vi "Read Parameter Spreadsheet.vi"(8 "error in (no error)":errorcluster) -> (0 "error out":errorcluster, 1 "Constraints":string[](array[string]), 2 "Types":string[](array[string]), 3 "Names":string[](array[string]), 5 "EnumVals":i32[](array[numeric]))   [LabVIEW 2020, in "Camera.lvlib"]
uses:
  Camera.lvlib
  <vilib>/Utility/file.llb/Read Delimited Spreadsheet (string).vi
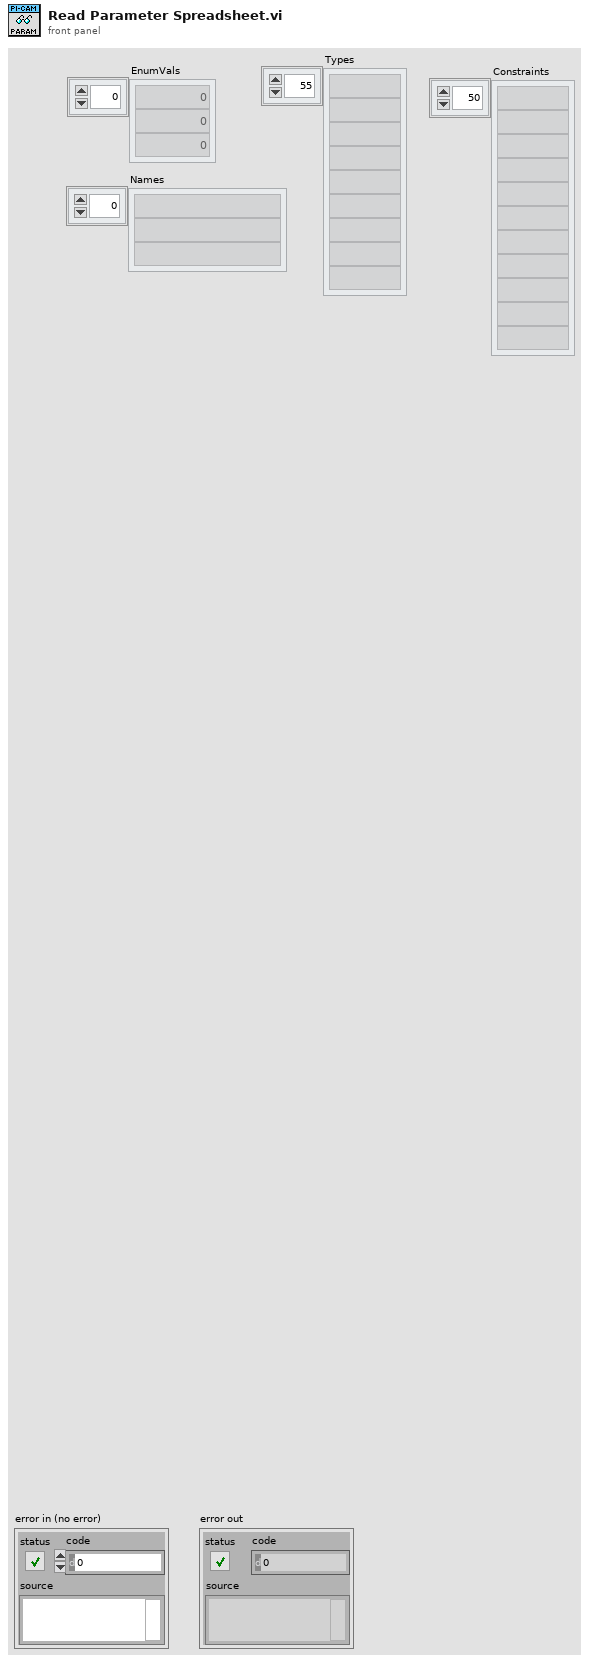
[diagram p1: front panel]
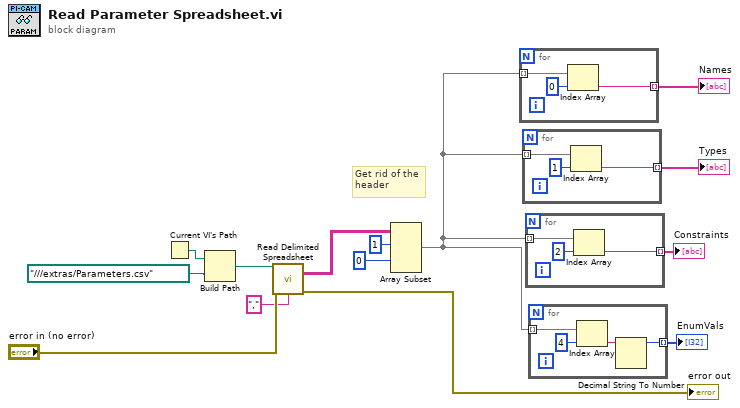
[diagram p0: block diagram]
diagram:
  # "Get rid of the\nheader"
  n1 = Current VI's Path() -> (path=w3:path)
  n2 = Build Path(base path=w3, name or relative path=path "../../../extras/Parameters.csv" ("file path (dialog if empty)")) -> (appended path=w4:path)
  n3 = call-poly <vilib>:"Read Delimited Spreadsheet.vi"("file path (dialog if empty)"=w4, "error in (no error)"="error in (no error)", "delimiter (\\t)"="," ("delimiter (\\t)")) -> ("all rows"=w6:string[][], "error out"=→"error out":errorcluster)  [unwired: 7 in, 4 out]
  n4 = Array Subset(array=w6, index (row)=1, index (col)=0 ("disabled index (col)")) -> (w12:string[][])  [unwired: 2 in]
  n5 = for {
    tunnel: w12 -> [w17] mode=indexing
    tunnel: [w15] -> w9 mode=indexing
    n6 = Index Array(array=w17, index=0) -> (element=w15:string)
  }
  "Names" <- w9
  n7 = for {
    tunnel: w12 -> [w20] mode=indexing
    tunnel: [w18] -> w10 mode=indexing
    n8 = Index Array(array=w20, index=1) -> (element=w18:string)
  }
  "Types" <- w10
  n9 = for {
    tunnel: w12 -> [w23] mode=indexing
    tunnel: [w21] -> w11 mode=indexing
    n10 = Index Array(array=w23, index=2) -> (element=w21:string)
  }
  "Constraints" <- w11
  n11 = for {
    tunnel: w12 -> [w27] mode=indexing
    tunnel: [w24] -> w13 mode=indexing
    n12 = Index Array(array=w27, index=4) -> (element=w25:string)
    n13 = Decimal String To Number(string=w25) -> (number=w24:i32)  [unwired: 2 in, 1 out]
  }
  "EnumVals" <- w13
